vi "RunDuringExperiment.vi"() -> ()   [LabVIEW 2014]
uses:
  GlobalVars.vi
panel:
  in  "Motion Channel":dbl=1.0
  out "error out":errorcluster
  out "Calibration Parameters":dbl[][](array[numeric])
  in  "Invert Sign":bool=TRUE
  out "SutterControllerOpen":bool
  out "SutterControllerRef":refnum<vi>
  out "Reference Averaging":bool
  in  "Set Reference":bool
  in  "Reference Averaging Samples":i32=10 min=2 max=10000 step=1
  out "Semaphore Operation Error":errorcluster
  out "global_semaphore_md":T1
  out "Motion Detection Error":bool
  out "Restarted":bool=TRUE
  in  "Enable Calibration":bool
  in  "Analyze Nth Frames":i32=2 min=1 step=1
  out "Motion Computation Error":errorcluster
  out "Elements in Data Queue":i32
  in  "Position Shift Limit (Microns)":dbl=3.0 min=0.0
  out "Out of Limits":bool
  out "Z1":waveform(dbl)(graph)
  out "Y1":waveform(dbl)(graph)
  out "X1":waveform(dbl)(graph)
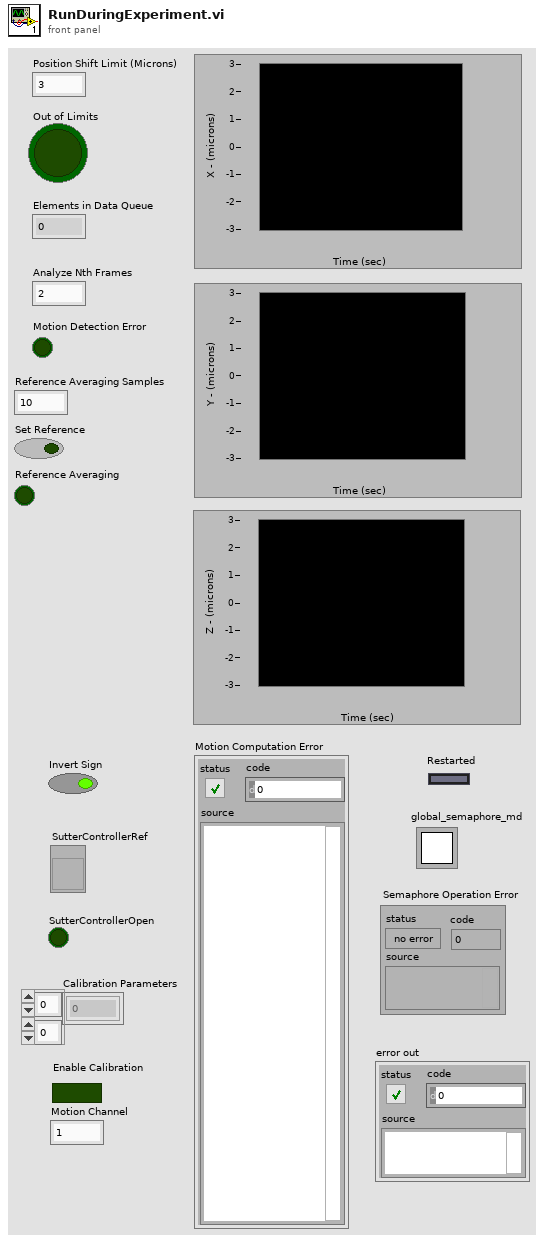
[diagram p1: front panel]
types:
  T1 = typedef "Semaphore RefNum" = refnum<k1>
  T2 = enum32{"Invalid", "Standard", "Closed", "Hidden", "Minimized", "Maximized"}
  T3 = enum16{"open", "replace", "create", "open or create", "replace or create", "replace or create with confirmation"}
  T4 = cluster{"gridsize":u16, "data":i32[][], "coordinates":i32[][], "settings":i32[], "settings_um":i32[], "needsreference":bool}
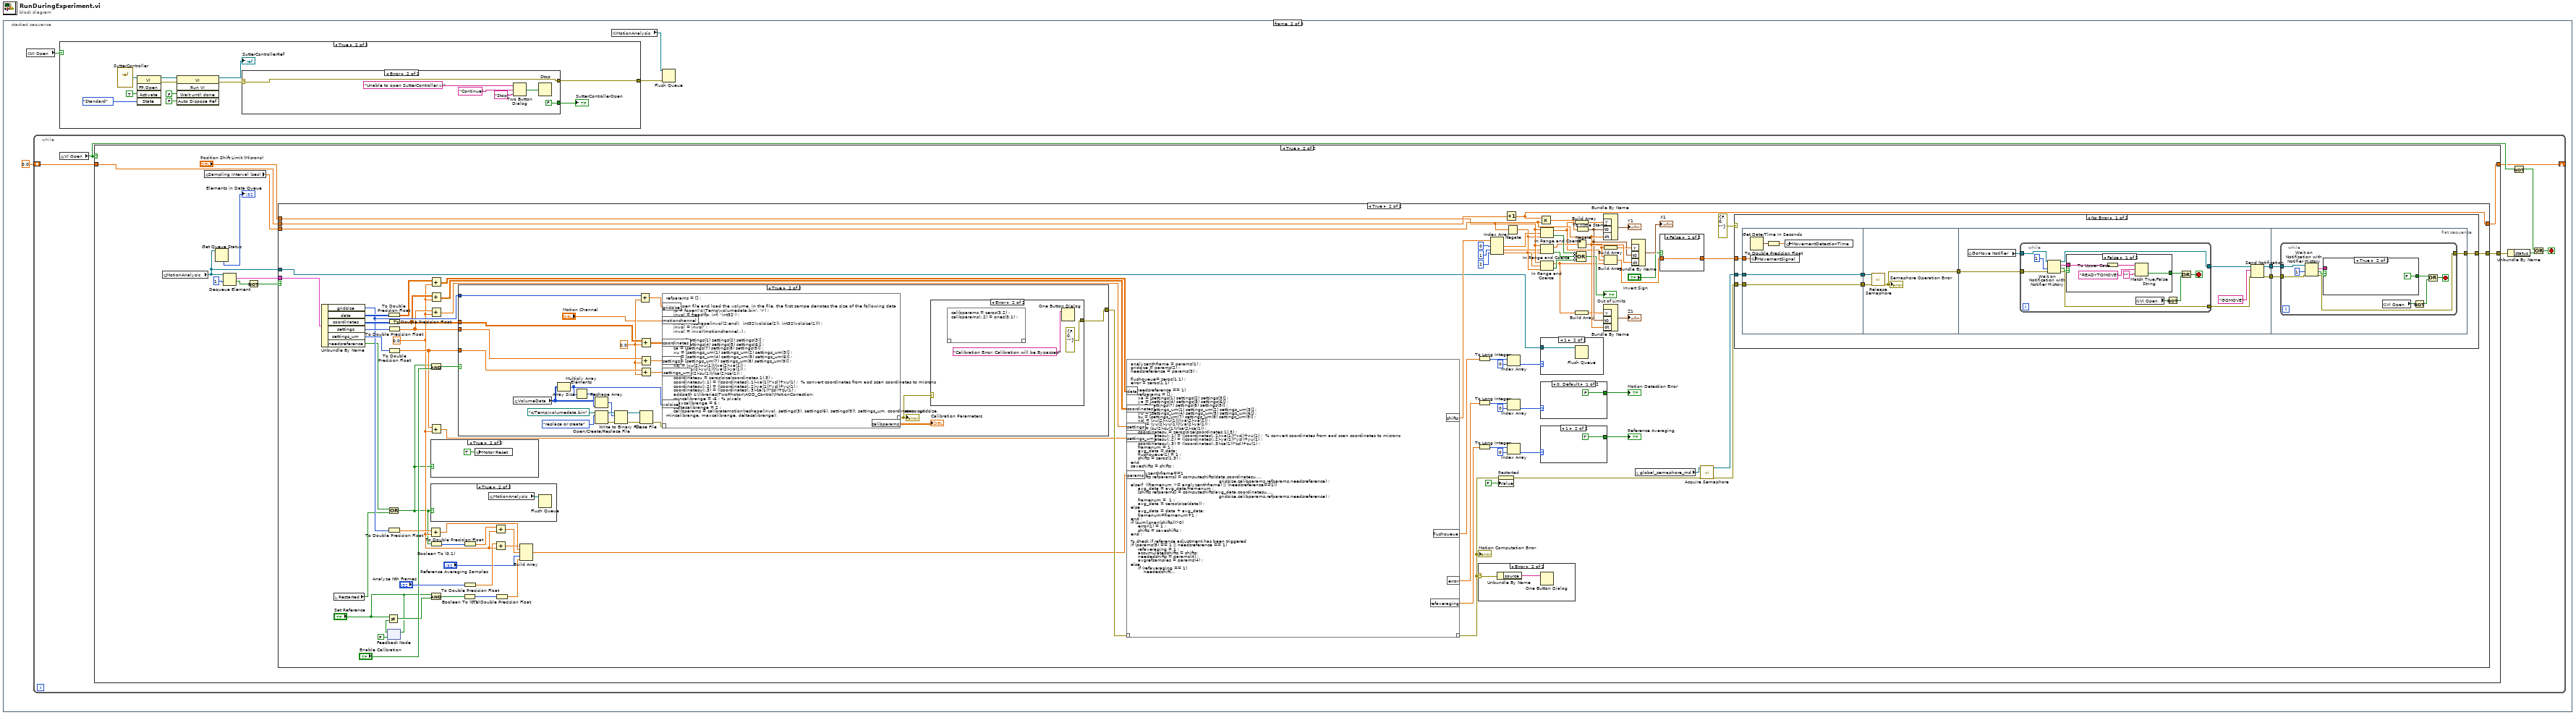
[diagram p0: block diagram]
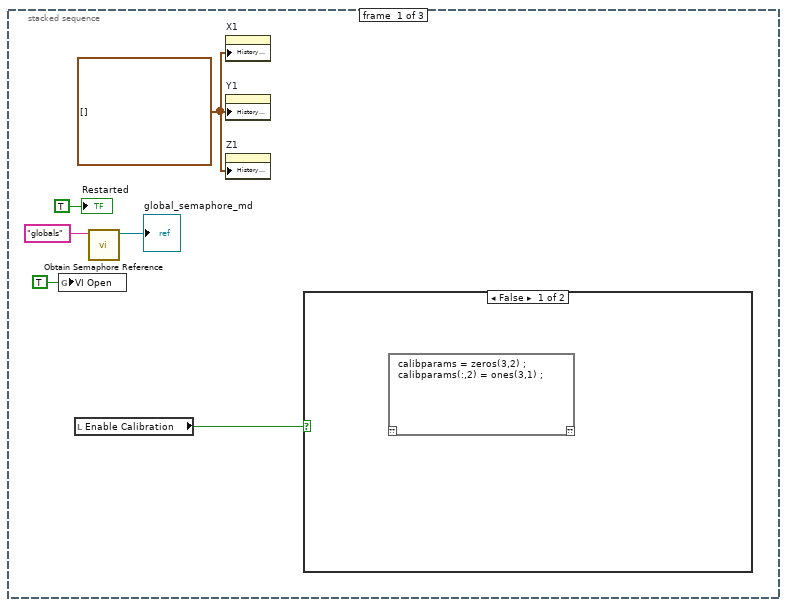
[diagram p2: hidden frame]
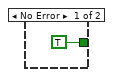
[diagram p5: hidden frame]
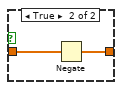
[diagram p9: hidden frame]
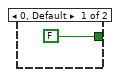
[diagram p11: hidden frame]
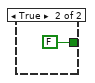
[diagram p13: hidden frame]
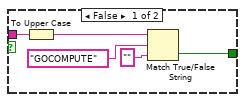
[diagram p14: hidden frame]
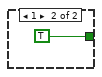
[diagram p16: hidden frame]
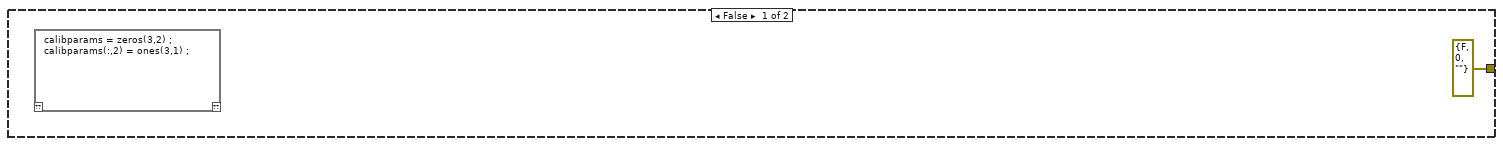
[diagram p18: hidden frame]
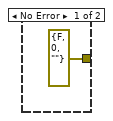
[diagram p19: hidden frame]
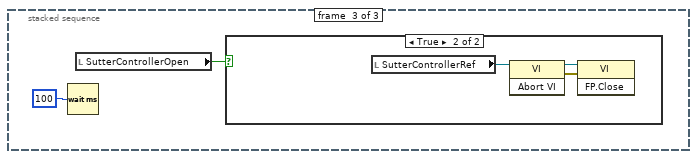
[diagram p20: hidden frame]
diagram:
  n1 = stacked-sequence {
    frame #0 {
      w5 = waveform(dbl)[] [] ("History Data")
      n2 = global write "GlobalVars.vi" "VI Open"(TRUE ("VI Open")) -> ()
      n3 = local read "Enable Calibration"() -> (w1:bool)
      n4 = call <vilib>:"Obtain Semaphore Reference.vi"("name (unnamed)"="globals") -> ("semaphore"=→"global_semaphore_md":T1)  [unwired: 4 in, 2 out]
      n5 = property on="X1" class="WFChart (strict)"("History Data"=w5) -> ()  [unwired: 2 in, 2 out]
      n6 = property on="Y1" class="WFChart (strict)"("History Data"=w5) -> ()  [unwired: 2 in, 2 out]
      n7 = property on="Z1" class="WFChart (strict)"("History Data"=w5) -> ()  [unwired: 2 in, 2 out]
      n8 = case shown="False" w1 {
        frame False {
          n9 = script code="calibparams = zeros(3,2) ;\ncalibparams(:,2) = ones(3,1) ;"() -> ()  [unwired: 1 in, 1 out]
        }
        frame True {
        }
      }
      "Restarted" <- TRUE ("Restarted")
    }
    frame #1 {
      n10 = global read "GlobalVars.vi" "VI Open"() -> (w9:bool)
      n11 = while {
        shift-right: [w33] -> _
        shift-left: 0.0 -> [w34]
        stop <- w31 stop-if-true
        n12 = global read "GlobalVars.vi" "VI Open"() -> (w35:bool)
        n13 = case shown="True" w35 {
          tunnel: w34 -> [w36 w44]
          tunnel: [w36 w43] -> w33
          tunnel: [_ w40] -> w29
          frame False {
          }
          frame True {
            n14 = global read "GlobalVars.vi" "MotionAnalysis"() -> (w41:refnum<queue>)
            n15 = global read "GlobalVars.vi" "Sampling Interval (sec)"() -> (w42:dbl)
            n16 = Get Queue Status(queue=w41) -> (# elements in queue=→"Elements in Data Queue":i32)  [unwired: 2 in, 7 out]
            n17 = Dequeue Element(queue=w41, timeout in ms (-1)=1) -> (element=w46:T4, timed out?=w39:bool)  [unwired: 1 in, 2 out]
            n18 = Not(x=w39) -> (.not. x?=w37:bool)
            n19 = case shown="True" w37 {
              tunnel: "Position Shift Limit (Microns)" -> [_ w124]
              tunnel: w46 -> [_ w137]
              tunnel: w42 -> [_ w139]
              tunnel: w44 -> [w48 w140]
              tunnel: [w48 w104] -> w43
              tunnel: w41 -> [_ w130]
              tunnel: [_ w52] -> w40
              frame False {
              }
              frame True {
                w112 = 0.0 ("y")
                n20 = Unbundle By Name(w137) -> ("gridsize"=w128:u16, "data"=w136:i32[][], "coordinates"=w135:i32[][], "settings"=w134:i32[], "settings_um"=w133:i32[], "needsreference"=w111:bool)
                n21 = local read "Restarted"() -> (w109:bool)
                n22 = To Double Precision Float(number=w136) -> (double precision float=w116:dbl[][])
                n23 = Or(x=w111, y=w109) -> (x .or. y?=w50:bool)
                n24 = To Double Precision Float(number=w128) -> (double precision float=w114:dbl)
                n25 = feedback-in #1("Set Reference") -> ()
                n26 = feedback #1(FALSE ("Set Reference")) -> (w63:bool)
                n27 = Not Equal?(x="Set Reference", y=w63) -> (x != y?=w61:bool)
                n28 = To Double Precision Float(number=w135) -> (double precision float=w118:dbl[][])
                n29 = To Double Precision Float(number=w134) -> (double precision float=w120:dbl[])
                n30 = To Double Precision Float(number=w133) -> (double precision float=w122:dbl[])
                n31 = Add(x=w114, y=w112) -> (x+y=w106:dbl)
                n32 = Add(x=w116, y=w112) -> (x+y=w115:dbl[][])
                n33 = Add(x=w118, y=w112) -> (x+y=w117:dbl[][])
                n34 = Add(x=w120, y=w112) -> (x+y=w119:dbl[])
                n35 = And(x=w50, y="Enable Calibration") -> (x .and. y?=w126:bool)
                n36 = Add(x=w122, y=w112) -> (x+y=w121:dbl[])
                n37 = Boolean To (0,1)(Boolean=w50) -> (0, 1=w132:i16)
                n38 = And(x="Set Reference", y=w61) -> (x .and. y?=w59:bool)
                n39 = case shown="True" w50 {
                  frame False {
                  }
                  frame True {
                    n40 = global write "GlobalVars.vi" "Motor Reset"(TRUE ("Motor Reset")) -> ()
                  }
                }
                n41 = case shown="True" w50 {
                  frame False {
                  }
                  frame True {
                    n42 = global read "GlobalVars.vi" "MotionAnalysis"() -> (w141:refnum<queue>)
                    n43 = Flush Queue(queue=w141) -> ()  [unwired: 1 in, 3 out]
                  }
                }
                n44 = case shown="True" w126 {
                  tunnel: w128 -> [_ w230]
                  tunnel: w118 -> [_ w232]
                  tunnel: w120 -> [_ w234]
                  tunnel: w122 -> [_ w236]
                  tunnel: [errorcluster {"status"=FALSE, "code"=0, "source"=""} ("error IO") w237] -> w125
                  frame False {
                    n45 = script code="calibparams = zeros(3,2) ;\ncalibparams(:,2) = ones(3,1) ;"() -> ()  [unwired: 1 in, 1 out]
                  }
                  frame True {
                    w229 = 0.0 ("y")
                    n46 = global read "GlobalVars.vi" "VolumeData"() -> (w222:i32[][])
                    n47 = Array Size(array=w222) -> (size(s)=w217:i32[])
                    n48 = Multiply Array Elements(1:w217) -> (0:w225:i32)
                    n49 = Reshape Array(w222, w225) -> (w219:i32[])
                    n50 = Open/Create/Replace File(file path (use dialog)=path "c:/Temp/volumedata.bin", operation (0:open)=T3."replace or create") -> (refnum out=w224:refnum<file>, error out=w220:errorcluster)  [unwired: 4 in, 1 out]
                    n51 = Write to Binary File(file (use dialog)=w224, data=w219, error in=w220) -> (refnum out=w223:refnum<file>, error out=w218:errorcluster)  [unwired: 3 in, 1 out]
                    n52 = Add(x=w230, y=w229) -> (x+y=w228:dbl)
                    n53 = Add(x=w232, y=w229) -> (x+y=w231:dbl[][])
                    n54 = Add(x=w234, y=w229) -> (x+y=w233:dbl[])
                    n55 = Add(x=w236, y=w229) -> (x+y=w235:dbl[])
                    n56 = Close File(refnum=w223, error in=w218) -> (error out=w221:errorcluster)  [unwired: 1 out]
                    n57 = script code="refparams = [] ;\n\n     % open file and load the volume, in the file, the first sampe denotes the size of the following data\n     fp = fopen('c:\\Temp\\volumedata.bin', 'r') ;\n     invol = fread(fp, inf, 'int32') ;\n     fclose(fp) ;\n     invol = reshape(invol(2:end),  int32(volsize(2)), int32(volsize(1))) ;\n     invol = invol' ;\n     invol = invol(motionchannel,:) ;\n\n     xa = [settings(1) settings(2) settings(3)] ;\n     ya = [settings(4) settings(5) settings(6)] ;\n     za = [settings(7) settings(8) settings(9)] ;\n     xu = [settings_um(1) settings_um(2) settings_um(3)] ;\n     yu = [settings_um(4) settings_um(5) settings_um(6)] ;\n     zu = [settings_um(7) settings_um(8) settings_um(9)] ;\n     xsl = (xu(2)-xu(1))/(xa(2)-xa(1)) ;\n     ysl = (yu(2)-yu(1))/(ya(2)-ya(1)) ;\n     zsl = (zu(2)-zu(1))/(za(2)-za(1)) ;\n     coordinatesu = zeros(size(coordinates,1),3) ;\n     coordinatesu(:,1) = ((coordinates(:,1)-xa(1))*xsl)+xu(1) ;  % convert coordinates from aod scan coordinates to microns\n     coordinatesu(:,2) = ((coordinates(:,2)-ya(1))*ysl)+yu(1) ;\n     coordinatesu(:,3) = ((coordinates(:,3)-za(1))*zsl)+zu(1) ;\n     addpath z:\\libraries\\TwoPhoton\\AOD_Control\\MotionCorrection;\n     mincalibrange = -6 ; % pixels\n     maxcalibrange = 6 ;\n     deltacalibrange = 2 ;\n     calibparams = calibratemotion(reshape(invol, settings(3), settings(6), settings(9)), settings_um, coordinatesu, gridsize, mincalibrange, maxcalibrange, deltacalibrange);"("??"=w221, "coordinates"=w231, "gridsize"=w228, "settings"=w233, "settings_um"=w235, "volsize"=w217, "motionchannel"="Motion Channel") -> ("??"=w238:errorcluster, "calibparams"=→"Calibration Parameters":dbl[][])
                    "error out" <- w238
                    n58 = case shown="Error" w238 {
                      tunnel: [errorcluster {"status"=FALSE, "code"=0, "source"=""} ("error IO") errorcluster {"status"=FALSE, "code"=0, "source"=""} ("error IO")] -> w237
                      frame No Error {
                      }
                      frame Error {
                        n59 = script code="calibparams = zeros(3,2) ;\ncalibparams(:,2) = ones(3,1) ;"() -> ()  [unwired: 1 in, 1 out]
                        n60 = One Button Dialog(message="Calibration Error: Calibration will be Bypassed") -> ()  [unwired: 1 in, 1 out]
                      }
                    }
                  }
                }
                n61 = Boolean To (0,1)(Boolean=w59) -> (0, 1=w62:i16)
                n62 = To Double Precision Float(number=w132) -> (double precision float=w123:dbl)
                n63 = To Double Precision Float(number="Analyze Nth Frames") -> (double precision float=w113:dbl)
                n64 = Add(x=w123, y=w112) -> (x+y=w108:dbl)
                n65 = Add(x=w113, y=w112) -> (x+y=w105:dbl)
                n66 = To Double Precision Float(number=w62) -> (double precision float=w64:dbl)
                n67 = Build Array(w105, w106, w108, "Reference Averaging Samples", w64) -> (w107:dbl[])
                n68 = script code="analyzenthframe = params(1) ;\ngridsize = params(2) ;\nneedsreference = params(3) ;\n\nflushqueue= zeros(1,1) ;\nerror = zeros(1,1)  ;\n\nif (needsreference == 1)\n     refparams = [] ;\n     xa = [settings(1) settings(2) settings(3)] ;\n     ya = [settings(4) settings(5) settings(6)] ;\n     za = [settings(7) settings(8) settings(9)] ;\n     xu = [settings_um(1) settings_um(2) settings_um(3)] ;\n     yu = [settings_um(4) settings_um(5) settings_um(6)] ;\n     zu = [settings_um(7) settings_um(8) settings_um(9)] ;\n     xsl = (xu(2)-xu(1))/(xa(2)-xa(1)) ;\n     ysl = (yu(2)-yu(1))/(ya(2)-ya(1)) ;\n     zsl = (zu(2)-zu(1))/(za(2)-za(1)) ;\n     coordinatesu = zeros(size(coordinates,1),3) ;\n     coordinatesu(:,1) = ((coordinates(:,1)-xa(1))*xsl)+xu(1) ;  % convert coordinates from aod scan coordinates to microns\n     coordinatesu(:,2) = ((coordinates(:,2)-ya(1))*ysl)+yu(1) ;\n     coordinatesu(:,3) = ((coordinates(:,3)-za(1))*zsl)+zu(1) ;\n     framenum = 1 ;\n     avg_data = data;\n     flushqueue(1) = 1 ;\n     shifts = zeros(1,3) ;\nend\nsaveshifts = shifts ;\n\nif analyzenthframe==1\n     [shifts refparams] = computeshifts(data,coordinatesu,...\n                                                             gridsize,calibparams,refparams,needsreference) ; \nelseif  ((framenum >= analyzenthframe) || (needsreference==1))\n     avg_data = avg_data/framenum ;\n     [shifts refparams] = computeshifts(avg_data,coordinatesu,...\n                                                             gridsize,calibparams,refparams,needsreference) ; \n     framenum =  1 ;\n     avg_data = zeros(size(data)) ;\nelse\n     avg_data = data + avg_data;\n     framenum=framenum+1 ;\nend ;\nif (sum(isnan(shifts))>0)\n     error(1) = 1 ;\n     shifts = saveshifts ;\nend ;\n\n% check if reference adjustment has been triggered\nif (params(5) == 1 || needsreference == 1)\n     refaveraging = 1 ;\n     accumulatedshifts = shifts;\n     neededshifts = params(4) ;\n     avgrefsamples = params(4) ;\nelse\n     if (refaveraging == 1)\n         neededshifts = neededshifts - 1 ;\n         if (neededshifts ~= 0)\n              accumulatedshifts = accumulatedshifts + shifts ;\n          else\n              refparams(3) = refparams(3)+accumulatedshifts(1)/avgrefsamples ;\n              refparams(5) = refparams(5)+accumulatedshifts(2)/avgrefsamples ;\n              refparams(7) = refparams(7)+accumulatedshifts(3)/avgrefsamples ;\n              refaveraging = 0 ;\n          end ;\n     end ;\nend ;"("??"=w125, "data"=w115, "coordinates"=w117, "settings"=w119, "settings_um"=w121, "params"=w107) -> ("??"=w110:errorcluster, "shifts"=w138:dbl[], "flushqueue"=w129:dbl[], "error"=w103:dbl[], "refaveraging"=w56:dbl[])
                "Motion Computation Error" <- w110
                n69 = To Long Integer(number=w129) -> (32bit integer=w102:i32[])
                n70 = To Long Integer(number=w103) -> (32bit integer=w97:i32[])
                n71 = To Long Integer(number=w56) -> (32bit integer=w58:i32[])
                n72 = case shown="Error" w110 {
                  selector: w110 -> [_ w213]
                  frame No Error {
                  }
                  frame Error {
                    n73 = Unbundle By Name(w213) -> ("source"=w212:string)
                    n74 = One Button Dialog(message=w212) -> ()  [unwired: 1 in, 1 out]
                  }
                }
                n75 = Index Array(array=w138, index #1=0 ("index"), index #2=1 ("index"), index #3=2 ("index")) -> (element #1=w81:dbl, element #2=w80:dbl, element #3=w79:dbl)
                n76 = property on="Restarted" class="Bool (strict)"(error in=w110, "Value"=FALSE ("Restarted")) -> (error out=w53:errorcluster)  [unwired: 1 in, 1 out]
                n77 = Increment(x=w140) -> (x+1=w104:dbl)
                n78 = Negate(x=w124) -> (-x=w66:dbl)
                n79 = Index Array(array=w102, index=0 ("index (row)")) -> (element=w101:i32)
                n80 = Index Array(array=w97, index=0) -> (element=w95:i32)
                n81 = Index Array(array=w58, index=0) -> (element=w55:i32)
                n82 = Multiply(x=w104, y=w139) -> (x*y=w83:dbl)
                n83 = In Range and Coerce(upper limit=w124, x=w81, lower limit=w66) -> (coerced(x)=w68:dbl, In Range?=w78:bool)
                n84 = In Range and Coerce(upper limit=w124, x=w80, lower limit=w66) -> (coerced(x)=w70:dbl, In Range?=w77:bool)
                n85 = In Range and Coerce(upper limit=w124, x=w79, lower limit=w66) -> (coerced(x)=w74:dbl, In Range?=w76:bool)
                n86 = case shown="1" w101 {
                  tunnel: w130 -> [_ w148]
                  frame 0, Default {
                  }
                  frame 1 {
                    n87 = Flush Queue(queue=w148) -> ()  [unwired: 1 in, 3 out]
                  }
                }
                n88 = case shown="0, Default" w95 {
                  tunnel: [FALSE ("Motion Detection Error") TRUE ("Motion Detection Error")] -> w98
                  frame 0, Default {
                  }
                  frame 1 {
                  }
                }
                "Motion Detection Error" <- w98
                n89 = case shown="1" w55 {
                  tunnel: [FALSE TRUE] -> w54
                  frame 0, Default {
                  }
                  frame 1 {
                  }
                }
                "Reference Averaging" <- w54
                n90 = Build Array(w68) -> (w84:dbl[])
                n91 = Negate(x=w70) -> (-x=w69:dbl)
                n92 = Build Array(w74) -> (w85:dbl[])
                n93 = To Time Stamp(1:w83) -> (0:w82:timestamp)
                n94 = Compound Arithmetic op=OR(invert w78, invert w77, invert w76) -> (→"Out of Limits":bool)
                n95 = Bundle By Name("Y"=w84, "t0"=w82, "dt"=w139) -> (→"Y1":waveform(dbl))  [unwired: 1 in]
                n96 = Bundle By Name("Y"=w85, "t0"=w82, "dt"=w139) -> (→"Z1":waveform(dbl))  [unwired: 1 in]
                n97 = Build Array(w69) -> (w88:dbl[])
                n98 = Build Array(w69, w68, w74) -> (w67:dbl[])
                n99 = Bundle By Name("Y"=w88, "t0"=w82, "dt"=w139) -> (→"X1":waveform(dbl))  [unwired: 1 in]
                n100 = local read "global_semaphore_md"() -> (w91:T1)
                n101 = case shown="False" "Invert Sign" {
                  tunnel: [w142 w144] -> w94
                  tunnel: w67 -> [w142 w143]
                  frame False {
                  }
                  frame True {
                    n102 = Negate(x=w143) -> (-x=w144:dbl[])
                  }
                }
                n103 = call <vilib>:"Acquire Semaphore.vi"("error in (no error)"=w53, "semaphore"=w91) -> ("error out"=w93:errorcluster, "semaphore out"=w92:T1)  [unwired: 3 in, 1 out]
                n104 = case shown="No Error" errorcluster {"status"=FALSE, "code"=0, "source"=""} ("error IO") {
                  tunnel: w94 -> [w157 _]
                  tunnel: w93 -> [w153 w209]
                  tunnel: w92 -> [w154 _]
                  tunnel: [w152 w209] -> w52
                  frame No Error {
                    n105 = flat-sequence {
                      tunnel: w157 -> [w162]
                      tunnel: w154 -> [w159]
                      tunnel: [w159] -> w151
                      tunnel: w153 -> [w158]
                      tunnel: [w158] -> w150
                      tunnel: w151 -> [w165]
                      tunnel: w150 -> [w164]
                      tunnel: [w163] -> w149
                      tunnel: [w171] -> w156
                      tunnel: [w170] -> w155
                      tunnel: w149 -> [w167]
                      tunnel: w156 -> [w192]
                      tunnel: w155 -> [w191]
                      tunnel: [w190] -> w152
                      frame #0 {
                        n106 = Get Date/Time In Seconds() -> (seconds since 1Jan1904=w161:timestamp)
                        n107 = global write "GlobalVars.vi" "MovementSignal"(w162) -> ()
                        n108 = To Double Precision Float(number=w161) -> (double precision float=w160:dbl)
                        n109 = global write "GlobalVars.vi" "MovementDetectionTime"(w160) -> ()
                      }
                      frame #1 {
                        n110 = call <vilib>:"Release Semaphore.vi"("error in (no error)"=w164, "semaphore"=w165) -> ("error out"=w163:errorcluster)  [unwired: 4 in, 1 out]
                        "Semaphore Operation Error" <- w163
                      }
                      frame #2 {
                        n111 = global read "GlobalVars.vi" "GoMove Notifier"() -> (w166:refnum<notifier>)
                        n112 = while {
                          tunnel: w166 -> [w181]
                          tunnel: [w180] -> w168
                          tunnel: w167 -> [w179]
                          tunnel: [w178] -> w169
                          stop <- w176 stop-if-true
                          n113 = Wait on Notification with Notifier History(0:w181, 2:1 ("timeout in ms (-1)"), 3:w179) -> (8:w180:refnum<notifier>, 9:w182:string, 10:w183:bool, 11:w178:errorcluster)  [unwired: 1 in]
                          n114 = case shown="False" w183 {
                            tunnel: w182 -> [w185 _]
                            tunnel: [w184 FALSE ("selection")] -> w177
                            frame False {
                              n115 = To Upper Case(1:w185) -> (0:w188:string)
                              n116 = Match True/False String(2:"" ("false string"), 3:"READYTOMOVE" ("true string"), 4:w188) -> (0:w184:bool)  [unwired: 1 out]
                            }
                            frame True {
                            }
                          }
                          n117 = global read "GlobalVars.vi" "VI Open"() -> (w175:bool)
                          n118 = Not(x=w175) -> (.not. x?=w174:bool)
                          n119 = Or(x=w177, y=w174) -> (x .or. y?=w176:bool)
                        }
                        n120 = Send Notification(notification="GOMOVE", notifier=w168, error in (no error)=w169) -> (notifier out=w171:refnum<notifier>, error out=w170:errorcluster)
                      }
                      frame #3 {
                        n121 = while {
                          tunnel: w192 -> [w202]
                          tunnel: w191 -> [w201]
                          tunnel: [w197] -> w190
                          stop <- w195 stop-if-true
                          n122 = Wait on Notification with Notifier History(0:w202, 2:1 ("timeout in ms (-1)"), 3:w201) -> (9:w198:string, 10:w199:bool, 11:w197:errorcluster)  [unwired: 1 in, 1 out]
                          n123 = case shown="True" w199 {
                            tunnel: w198 -> [w207 _]
                            tunnel: [w204 FALSE ("selection")] -> w196
                            frame False {
                              n124 = To Upper Case(1:w207) -> (0:w206:string)
                              n125 = Match True/False String(2:"" ("false string"), 3:"GOCOMPUTE" ("true string"), 4:w206) -> (0:w204:bool)  [unwired: 1 out]
                            }
                            frame True, Default {
                            }
                          }
                          n126 = global read "GlobalVars.vi" "VI Open"() -> (w193:bool)
                          n127 = Not(x=w193) -> (.not. x?=w194:bool)
                          n128 = Or(x=w196, y=w194) -> (x .or. y?=w195:bool)
                        }
                      }
                    }
                  }
                  frame Error {
                  }
                }
              }
            }
          }
        }
        n129 = Unbundle By Name(w29) -> ("status"=w30:bool)
        n130 = Not(x=w35) -> (.not. x?=w32:bool)
        n131 = Or(x=w32, y=w30) -> (x .or. y?=w31:bool)
      }
      n132 = case shown="True" w9 {
        tunnel: [_ w11] -> w7
        frame False {
        }
        frame True {
          n133 = vi-ref "SutterController.vi"() -> (w21:refnum<vi>)
          n134 = invoke class="VI" method="FP.Open"(reference=w21, "Activate"=TRUE ("Wait Until Done"), "State"=T2."Standard") -> (reference out=w18:refnum<vi>, error out=w17:errorcluster)  [unwired: 2 in, 3 out]
          n135 = invoke class="VI" method="Run VI"(reference=w18, error in=w17, "Wait until done"=FALSE ("Wait Until Done"), "Auto Dispose Ref"=FALSE ("Auto Dispose Reference")) -> (reference out=→"SutterControllerRef":refnum<vi>, error out=w12:errorcluster)  [unwired: 1 in, 3 out]
          n136 = case shown="Error" w12 {
            selector: w12 -> [_ w23]
            tunnel: [TRUE ("SutterControllerOpen") FALSE ("SutterControllerOpen")] -> w13
            tunnel: [_ w23] -> w11
            frame No Error {
            }
            frame Error {
              n137 = Two Button Dialog(message="Unable to open SutterController.vi", 1:"Stop" ("F button name (\"Cancel\")"), 2:"Continue" ("T button name (\"OK\")")) -> (T button?=w25:bool)
              n138 = Stop(stop? (T)=w25) -> ()
            }
          }
          "SutterControllerOpen" <- w13
        }
      }
      n139 = global read "GlobalVars.vi" "MotionAnalysis"() -> (w8:refnum<queue>)
      n140 = Flush Queue(queue=w8, error in (no error)=w7) -> ()  [unwired: 3 out]
    }
    frame #2 {
      n141 = Wait (ms)(milliseconds to wait=u32 100) -> ()  [unwired: 1 out]
      n142 = local read "SutterControllerOpen"() -> (w243:bool)
      n143 = case shown="True" w243 {
        frame False {
        }
        frame True {
          n144 = local read "SutterControllerRef"() -> (w244:refnum<vi>)
          n145 = invoke class="VI" method="Abort VI"(reference=w244) -> (reference out=w246:refnum<vi>, error out=w245:errorcluster)  [unwired: 2 in, 1 out]
          n146 = invoke class="VI" method="FP.Close"(reference=w246, error in=w245) -> ()  [unwired: 1 in, 3 out]
        }
      }
    }
  }
